vi "Low Gear Calibrations.vi"() -> ()   [LabVIEW 2016]
panel:
  in  "Low Gear Calibrations File Location":path=path "C:/ni-rt/startup/LowGearCalibrations.txt"
  out "Right Drive Integral Gain Low Gear":dbl
  out "Right Drive Derivative Low Gear":dbl
  out "Right Drive Feed-Forward Gain Low Gear":dbl
  out "Left Drive Derivative Gain Low Gear":dbl
  out "Left Drive Feed-Forward Gain Low Gear":dbl
  out "Right Drive Proportional Gain Low Gear":dbl
  out "Max RPM Low Gear":dbl
  out "Left Drive Proportional Gain Low Gear":dbl
  out "Left Drive Integral Gain Low Gear":dbl
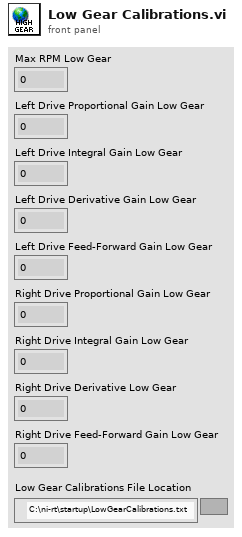
[diagram p1: front panel]
diagram:
